vi "Prop Control Interface (Main).vi"() -> ()   [LabVIEW 2013]
uses:
  Common/State Machine.ctl
panel:
  out "Training Data":i32[][](array[numeric])
  out "Increment?":bool
  out "Sensor 4":T1(graph)
  out "Sensor 3":T1(graph)
  out "Sensor 2":T1(graph)
  in  "Frequency":u8(ring)=1 items=["CHAN0", "CHAN1", "CHAN2", "CHAN3", "CHAN4", "CHAN5"]
  in  "Threshold":u16=2047
  out "Readback":u8[](array[numeric])
  out "VISA Port":refnum<visa-resource-name>="COM4"
  out "baud rate":u32=921600
  out "data queue":refnum<queue>
  out "User Message":string
  out "MagPosSlider":dbl(slide) caption="Magnet Position" min=0.0 max=15.0 step=0.5 scale=0.0..15.0
  out "eTDS Connected?":bool
  out "Buffer":i32[][](array[numeric])
  out "Sensor 1":T1(graph)
  in  "Exit":bool
  in  "Start":bool
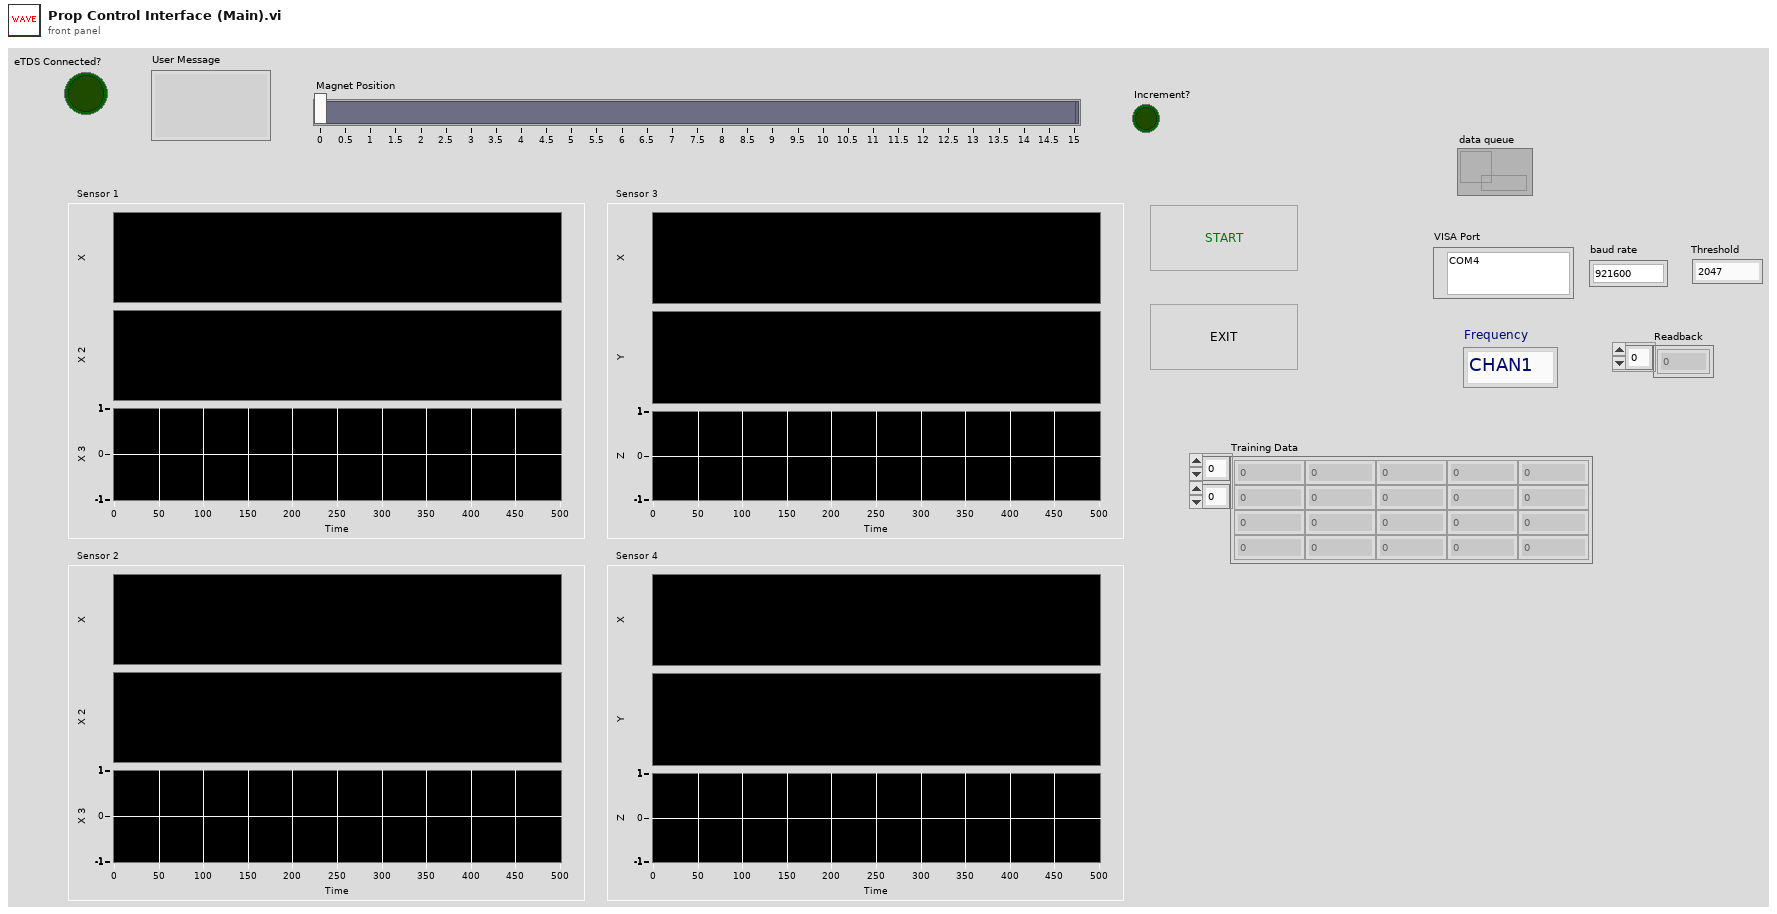
[diagram p1: front panel]
types:
  T1 = cluster{"Sensor 1[0]":i32, "Sensor 1[1]":i32, "Sensor 1[2]":i32}
  T2 = typedef "State Machine.ctl" = enum16{"Start", "Increment Slider", "Read Data", "Training SSP", "Stop"}
  T3 = enum8{"Enabled", "Disabled", "Disabled and Grayed Out"}
  T4 = cluster{"Sensor 1[0]":i32, "Sensor 1[1]":i32, "Sensor 1[2]":i32}[]
  T5 = cluster{"Sensor 4[0]":i32, "Sensor 4[1]":i32, "Sensor 4[2]":i32}
  T6 = cluster{"Sensor 3[0]":i32, "Sensor 3[1]":i32, "Sensor 3[2]":i32}
  T7 = cluster{"Sensor 2[0]":i32, "Sensor 2[1]":i32, "Sensor 2[2]":i32}
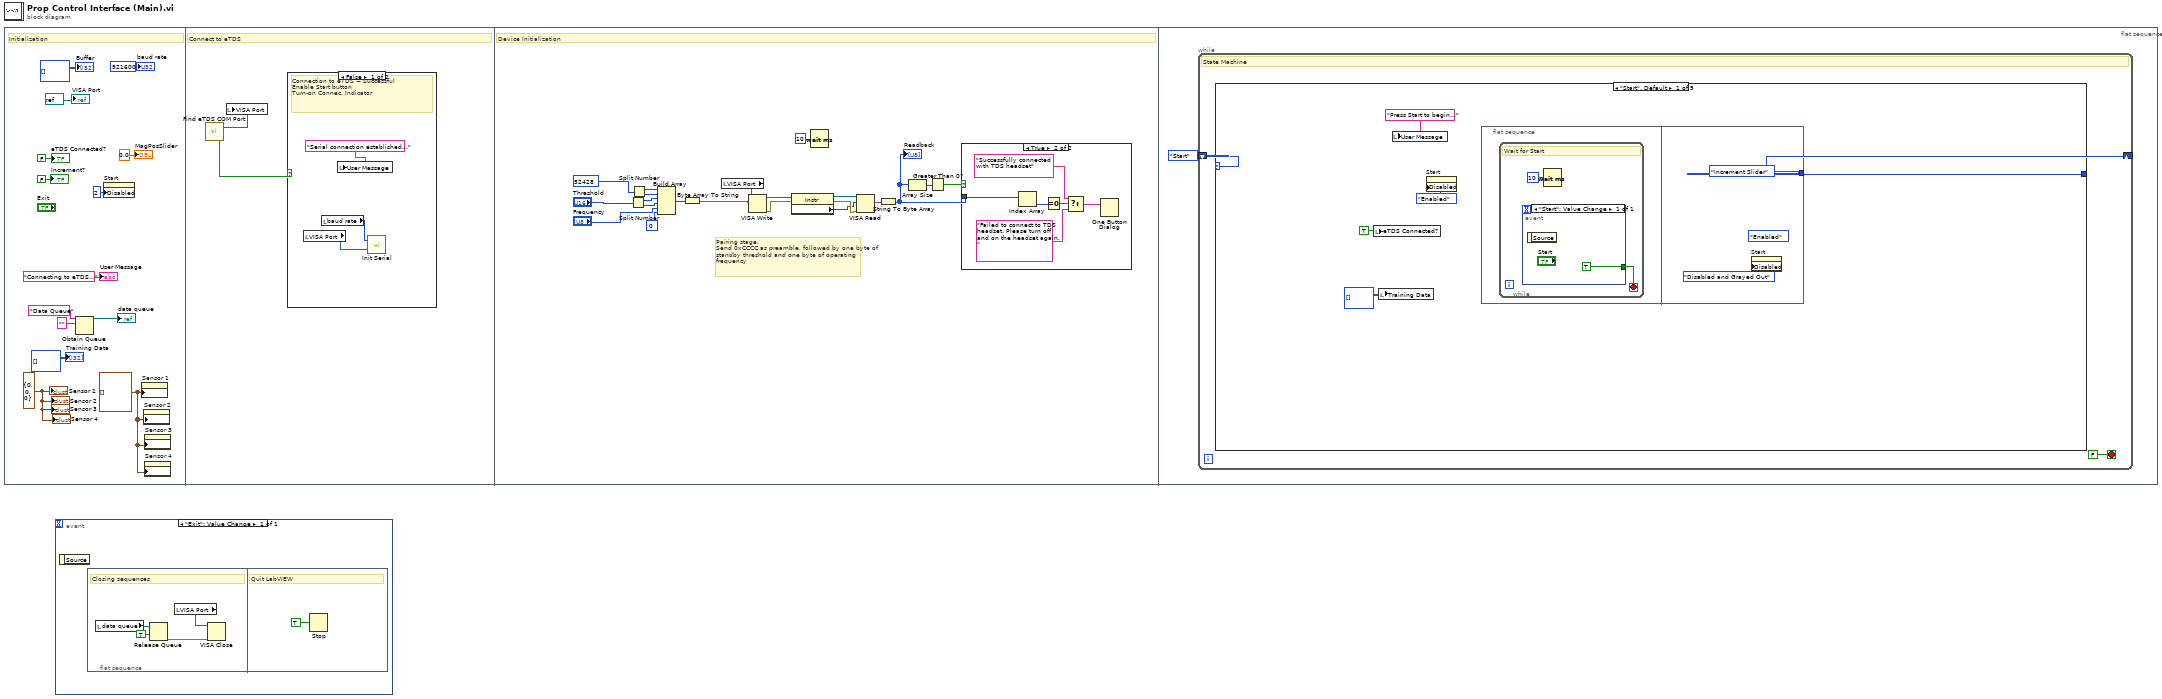
[diagram p0: block diagram]
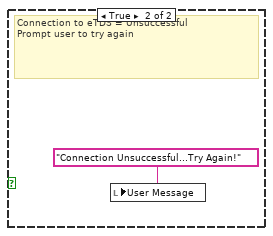
[diagram p2: hidden frame]
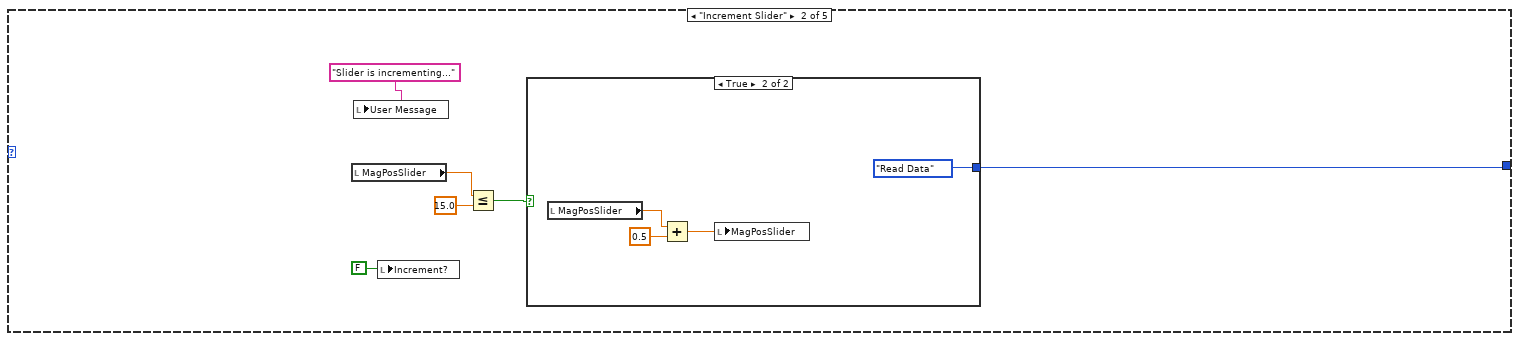
[diagram p4: hidden frame]
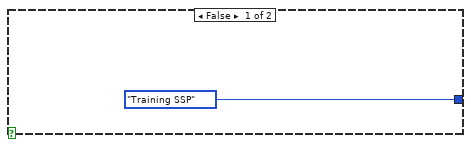
[diagram p5: hidden frame]
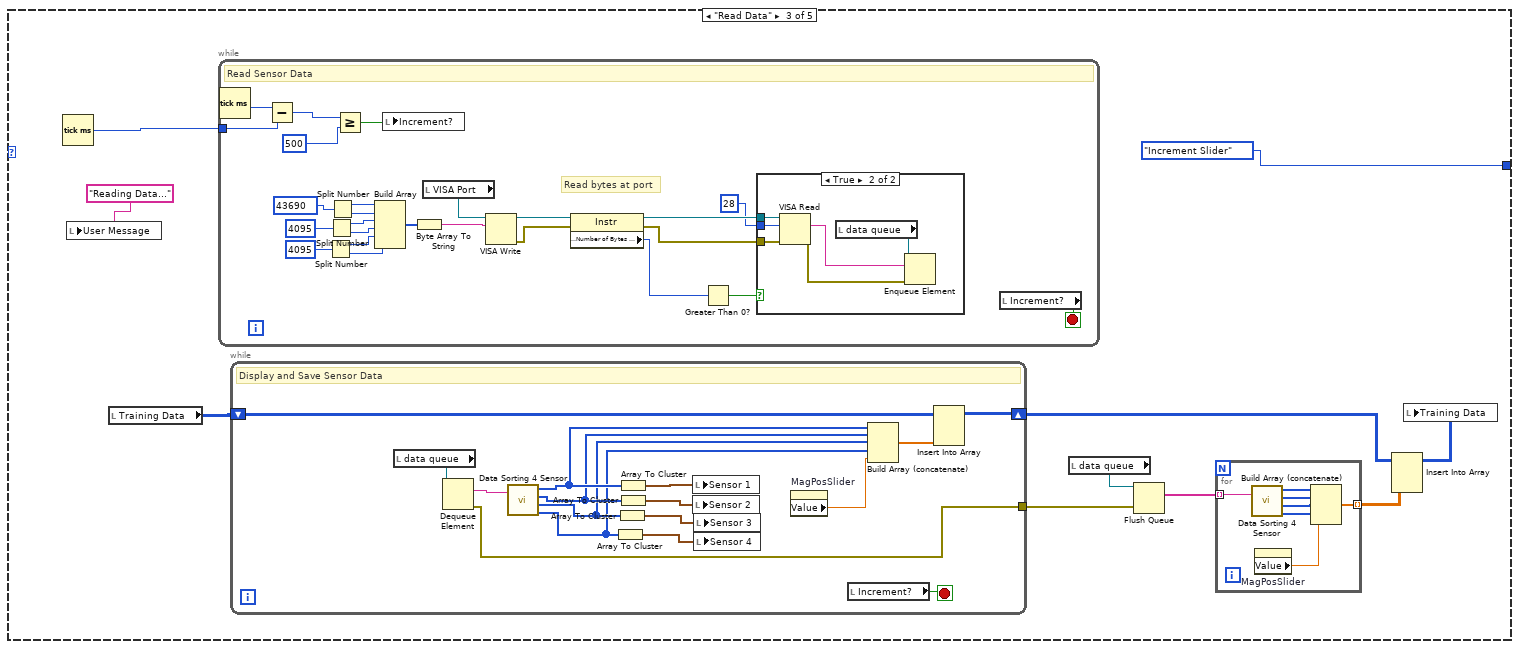
[diagram p6: hidden frame]
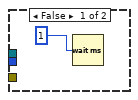
[diagram p7: hidden frame]
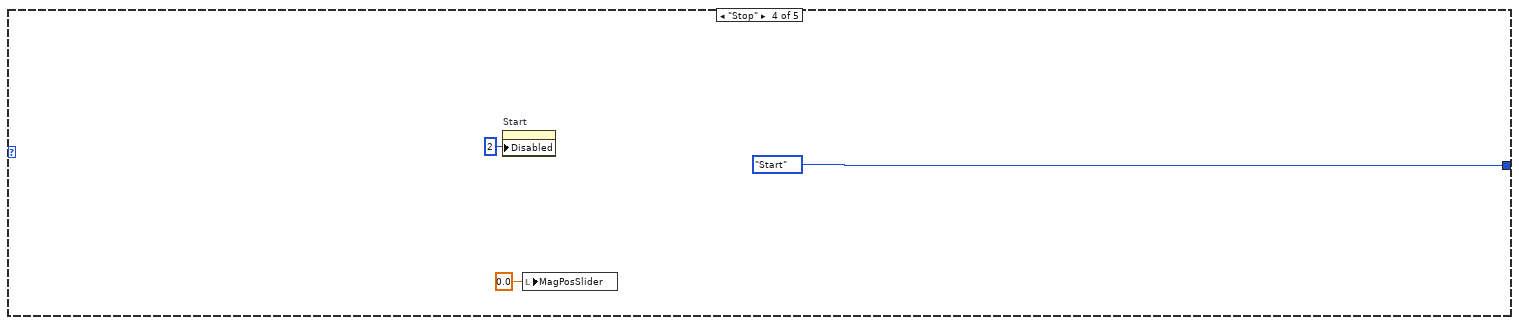
[diagram p8: hidden frame]
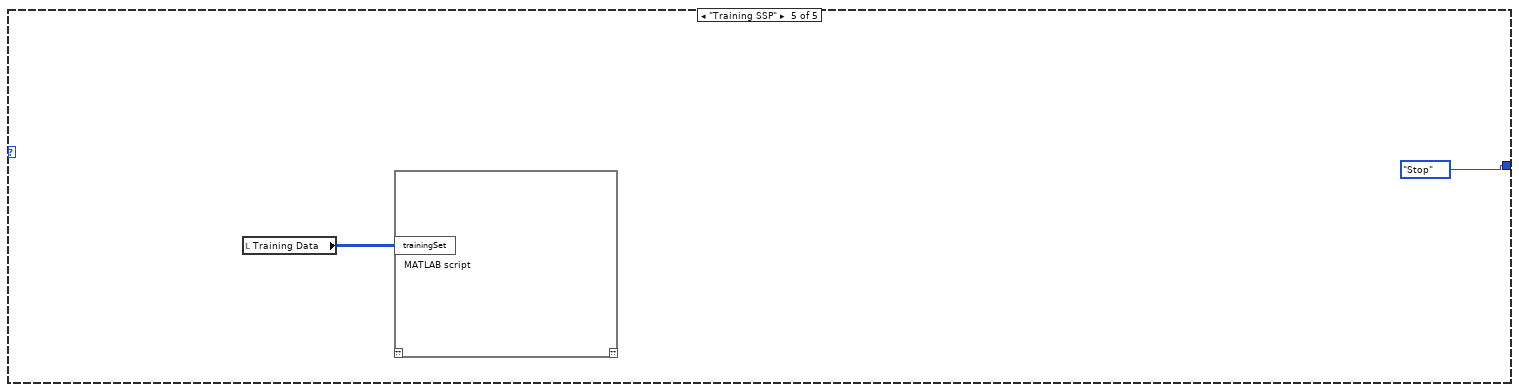
[diagram p9: hidden frame]
diagram:
  n1 = flat-sequence {
    frame #0 {
      w3 = T4 [] ("History Data")
      w4 = T1 {"Sensor 1[0]"=0, "Sensor 1[1]"=0, "Sensor 1[2]"=0} ("Sensor 1")
      # "Initialization"
      n2 = Obtain Queue(name (unnamed)="Data Queue" ("read buffer"), element data type="" ("read buffer")) -> (queue out=→"data queue":refnum<queue>)  [unwired: 3 in, 2 out]
      n3 = property on="Start" class="Bool"("Disabled"=u8 2) -> ()  [unwired: 2 in, 2 out]
      n4 = property on="Sensor 1" class="WFChart (strict)"("History Data"=w3) -> ()  [unwired: 2 in, 2 out]
      n5 = property on="Sensor 2" class="WFChart (strict)"("History Data"=w3) -> ()  [unwired: 2 in, 2 out]
      n6 = property on="Sensor 3" class="WFChart (strict)"("History Data"=w3) -> ()  [unwired: 2 in, 2 out]
      n7 = property on="Sensor 4" class="WFChart (strict)"("History Data"=w3) -> ()  [unwired: 2 in, 2 out]
      "eTDS Connected?" <- FALSE ("eTDS Connected?")
      "Buffer" <- i32[][] [] ("initialized array")
      "VISA Port" <- refnum<visa-resource-name> refnum ("VISA Resource Name")
      "baud rate" <- u32 921600 ("baud rate")
      "MagPosSlider" <- 0.0 ("MagPosSlider")
      "User Message" <- "Connecting to eTDS..." ("User Message")
      "Sensor 1" <- w4
      "Sensor 4" <- w4
      "Sensor 2" <- w4
      "Sensor 3" <- w4
      "Increment?" <- FALSE ("Increment?")
      "Training Data" <- i32[][] [] ("Training Data")
    }
    frame #1 {
      # "Connect to eTDS"
      n8 = call "Find eTDS COM Port.vi"() -> ("USB port"=w15:refnum<visa-resource-name>, "None/Multiple Device(s)?"=w16:bool)  [unwired: 1 in]
      n9 = local write "VISA Port"(w15) -> ()
      n10 = case shown="False" w16 {
        frame False {
          # "Connection to eTDS = Successful \nEnable Start button\nTurn-on Connec. Indicator"
          n11 = local read "VISA Port"() -> (w18:refnum<visa-resource-name>)
          n12 = local read "baud rate"() -> (w17:u32)
          n13 = local write "User Message"("Serial connection established..." ("User Message")) -> ()
          n14 = call "Init Serial.vi"("VISA resource name"=w18, "baud rate"=w17) -> ()  [unwired: 2 out]
        }
        frame True {
          # "Connection to eTDS = Unsuccessful\nPrompt user to try again"
          n15 = local write "User Message"("Connection Unsuccessful...Try Again!" ("User Message")) -> ()
        }
      }
    }
    frame #2 {
      # "Pairing stage.\nSend 0xCCCC as preamble, followed by one byte of standby threshold and one byte of operating frequency"
      # "Device Initialization"
      n16 = Split Number(x="Threshold") -> (hi(x)=w34:u8, lo(x)=w35:u8)
      n17 = Split Number(x=u16 52428 ("ChnA")) -> (hi(x)=w33:u8, lo(x)=w32:u8)
      n18 = Build Array(w33, w32, w34, w35, "Frequency", u8 0 ("ChnA")) -> (w31:u8[])
      n19 = Byte Array To String(unsigned byte array=w31) -> (string=w27:string)
      n20 = local read "VISA Port"() -> (w21:refnum<visa-resource-name>)
      n21 = VISA Write(VISA resource name=w21, write buffer=w27) -> (VISA resource name out=w25:refnum<visa-resource-name>, error out=w24:errorcluster)  [unwired: 1 in, 1 out]
      n22 = property class="Instr"(reference=w25, error in=w24) -> (reference out=w39:refnum<visa-resource-name>, error out=w38:errorcluster, "Serial Settings:Number of Bytes at Serial Port"=w36:u32)
      n23 = Wait (ms)(milliseconds to wait=u32 10) -> ()  [unwired: 1 out]
      n24 = VISA Read(VISA resource name=w39, byte count=w36, error in (no error)=w38) -> (read buffer=w37:string)  [unwired: 3 out]
      n25 = String To Byte Array(string=w37) -> (unsigned byte array=w26:u8[])
      "Readback" <- w26
      n26 = Array Size(array=w26) -> (size(s)=w40:i32)
      n27 = Greater Than 0?(x=w40) -> (x > 0?=w41:bool)
      n28 = case shown="True" w41 {
        tunnel: w26 -> [_ w43]
        frame False {
        }
        frame True {
          n29 = Index Array "Index Array"(array=w43) -> (element=w44:u8)  [unwired: 1 in]
          n30 = Equal To 0?(x=w44) -> (x = 0?=w42:bool)
          n31 = Select(t="Successfully connected with TDS headset", s=w42, f="Failed to connect to TDS headset. Please turn off and on the headset again.") -> (s? t:f=w47:string)
          n32 = One Button Dialog(message=w47) -> ()  [unwired: 1 in, 1 out]
        }
      }
    }
    frame #3 {
      n33 = while {
        shift-right: [w50] -> _
        shift-left: State_Machine."Start" -> [w49]
        stop <- FALSE stop-if-true
        # "State Machine"
        n34 = case shown="\"Start\", Default" w49 {
          tunnel: [w55 w65 State_Machine."Increment Slider" State_Machine."Start" State_Machine."Stop"] -> w50
          frame "Start", Default {
            n35 = local write "eTDS Connected?"(TRUE ("eTDS Connected?")) -> ()
            n36 = local write "Training Data"(i32[][] [] ("Training Data")) -> ()
            n37 = local write "User Message"("Press Start to begin..." ("User Message")) -> ()
            n38 = property on="Start" class="Bool"("Disabled"=T3."Enabled") -> ()  [unwired: 2 in, 2 out]
            n39 = flat-sequence {
              tunnel: [State_Machine."Increment Slider"] -> w55
              frame #0 {
                n40 = while {
                  stop <- w57 stop-if-true
                  # "Wait for Start"
                  n41 = event shown="[0] \"Start\": Value Change" {
                    selector: _ -> [_]
                    dyn-events: _ -> [_]
                    timeout: _ -> [_]
                    tunnel: [TRUE] -> w57
                    event "Start": Value Change {
                      n42 = event-data() -> ()  [unwired: 1 in, 1 out]
                    }
                  }
                  n43 = Wait (ms)(milliseconds to wait=u32 10) -> ()  [unwired: 1 out]
                }
              }
              frame #1 {
                (unwired) T3."Enabled" ("Disabled")
                n44 = property on="Start" class="Bool"("Disabled"=T3."Disabled and Grayed Out") -> ()  [unwired: 2 in, 2 out]
              }
            }
          }
          frame "Increment Slider" {
            n45 = local read "MagPosSlider"() -> (w67:dbl)
            n46 = local write "User Message"("Slider is incrementing..." ("User Message")) -> ()
            n47 = local write "Increment?"(FALSE ("Increment?")) -> ()
            n48 = Less Or Equal?(x=w67, y=15.0) -> (x <= y?=w63:bool)
            n49 = case shown="True" w63 {
              tunnel: [State_Machine."Training SSP" State_Machine."Read Data"] -> w65
              frame False {
              }
              frame True {
                n50 = local read "MagPosSlider"() -> (w71:dbl)
                n51 = Add(x=w71, y=0.5) -> (x+y=w70:dbl)
                n52 = local write "MagPosSlider"(w70) -> ()
              }
            }
          }
          frame "Read Data" {
            n53 = Tick Count (ms)() -> (millisecond timer value=w81:u32)
            n54 = local write "User Message"("Reading Data..." ("User Message")) -> ()
            n55 = local read "Training Data"() -> (w74:i32[][])
            n56 = while {
              tunnel: w81 -> [w110]
              stop <- w106 stop-if-true
              # "Read bytes at port"
              # "Read Sensor Data"
              n57 = Tick Count (ms)() -> (millisecond timer value=w111:u32)
              n58 = Subtract(x=w111, y=w110) -> (x-y=w109:u32)
              n59 = Split Number(x=u16 4095 ("ChnA")) -> (hi(x)=w117:u8, lo(x)=w116:u8)
              n60 = Split Number(x=u16 4095 ("ChnA")) -> (hi(x)=w122:u8, lo(x)=w123:u8)
              n61 = Split Number(x=u16 43690 ("ChnA")) -> (hi(x)=w121:u8, lo(x)=w120:u8)
              n62 = Greater Or Equal?(x=w109, y=u32 500 ("milliseconds to wait")) -> (x >= y?=w107:bool)
              n63 = Build Array(w121, w120, w122, w123, w117, w116) -> (w119:u8[])
              n64 = local write "Increment?"(w107) -> ()
              n65 = Byte Array To String(unsigned byte array=w119) -> (string=w118:string)
              n66 = local read "VISA Port"() -> (w112:refnum<visa-resource-name>)
              n67 = VISA Write(VISA resource name=w112, write buffer=w118) -> (VISA resource name out=w125:refnum<visa-resource-name>, error out=w124:errorcluster)  [unwired: 1 in, 1 out]
              n68 = property class="Instr"(reference=w125, error in=w124) -> (reference out=w129:refnum<visa-resource-name>, error out=w130:errorcluster, "Serial Settings:Number of Bytes at Serial Port"=w127:u32)
              n69 = Greater Than 0?(x=w127) -> (x > 0?=w128:bool)
              n70 = case shown="True" w128 {
                tunnel: w129 -> [_ w136]
                tunnel: w130 -> [_ w137]
                tunnel: u32 28 -> [_ w135]
                frame False {
                  n71 = Wait (ms)(milliseconds to wait=1) -> ()  [unwired: 1 out]
                }
                frame True {
                  n72 = VISA Read(VISA resource name=w136, byte count=w135, error in (no error)=w137) -> (read buffer=w134:string, error out=w133:errorcluster)  [unwired: 2 out]
                  n73 = local read "data queue"() -> (w132:refnum<queue>)
                  n74 = Enqueue Element(queue=w132, element=w134, error in (no error)=w133) -> ()  [unwired: 4 out]
                }
              }
              n75 = local read "Increment?"() -> (w106:bool)
            }
            n76 = while {
              shift-right: [w92] -> w76
              shift-left: w74 -> [w93]
              tunnel: [w90] -> w79
              stop <- w99 stop-if-true
              # "Display and Save Sensor Data"
              n77 = local read "data queue"() -> (w105:refnum<queue>)
              n78 = Dequeue Element(queue=w105) -> (element=w104:string, error out=w90:errorcluster)  [unwired: 1 in, 3 out]
              n79 = call "Data Sorting 4 Sensor.vi"("Data_Input"=w104) -> ("Sensor 1"=w98:i32[], "Sensor 2"=w97:i32[], "Sensor 3"=w96:i32[], "Sensor 4"=w95:i32[])  [unwired: 3 out]
              n80 = Array To Cluster(array=w95) -> (cluster=w100:T5)
              n81 = Array To Cluster(array=w96) -> (cluster=w101:T6)
              n82 = Array To Cluster(array=w98) -> (cluster=w103:T1)
              n83 = Array To Cluster(array=w97) -> (cluster=w102:T7)
              n84 = local write "Sensor 1"(w103) -> ()
              n85 = local write "Sensor 2"(w102) -> ()
              n86 = local write "Sensor 3"(w101) -> ()
              n87 = local write "Sensor 4"(w100) -> ()
              n88 = property on="MagPosSlider" class="Slide (strict)"() -> ("Value"=w91:dbl)  [unwired: 2 in, 2 out]
              n89 = local read "Increment?"() -> (w99:bool)
              n90 = Build Array (concatenate)(w98, w97, w96, w95, w91) -> (w94:dbl[])
              n91 = Insert Into Array(array=w93, new element=w94) -> (w92:i32[][])  [unwired: 2 in]
            }
            n92 = local read "data queue"() -> (w80:refnum<queue>)
            n93 = Flush Queue(queue=w80, error in (no error)=w79) -> (remaining elements=w78:string[])  [unwired: 2 out]
            n94 = for {
              tunnel: w78 -> [w89] mode=indexing
              tunnel: [w83] -> w77 mode=indexing
              n95 = call "Data Sorting 4 Sensor.vi"("Data_Input"=w89) -> ("Sensor 1"=w88:i32[], "Sensor 2"=w87:i32[], "Sensor 3"=w86:i32[], "Sensor 4"=w85:i32[])  [unwired: 3 out]
              n96 = property on="MagPosSlider" class="Slide (strict)"() -> ("Value"=w84:dbl)  [unwired: 2 in, 2 out]
              n97 = Build Array (concatenate)(w88, w87, w86, w85, w84) -> (w83:dbl[])
            }
            n98 = Insert Into Array(array=w76, new element=w77) -> (w75:i32[][])  [unwired: 2 in]
            n99 = local write "Training Data"(w75) -> ()
          }
          frame "Stop" {
            n100 = property on="Start" class="Bool"("Disabled"=u8 2) -> ()  [unwired: 2 in, 2 out]
            n101 = local write "MagPosSlider"(0.0 ("MagPosSlider")) -> ()
          }
          frame "Training SSP" {
            n102 = local read "Training Data"() -> (w142:i32[][])
            n103 = script code="MATLAB script"("trainingSet"=w142) -> ()  [unwired: 1 in, 1 out]
          }
        }
      }
    }
  }
  n104 = event shown="[0] \"Exit\": Value Change" {
    selector: _ -> [_]
    dyn-events: _ -> [_]
    timeout: _ -> [_]
    event "Exit": Value Change {
      n105 = event-data() -> ()  [unwired: 1 in, 1 out]
      n106 = flat-sequence {
        frame #0 {
          # "Closing sequences"
          n107 = local read "data queue"() -> (w145:refnum<queue>)
          n108 = Release Queue(queue=w145, force destroy? (F)=TRUE) -> (error out=w144:errorcluster)  [unwired: 1 in, 2 out]
          n109 = local read "VISA Port"() -> (w146:refnum<visa-resource-name>)
          n110 = VISA Close(VISA resource name=w146, error in (no error)=w144) -> ()  [unwired: 1 out]
        }
        frame #1 {
          # "Quit LabVIEW"
          n111 = Stop(stop? (T)=TRUE ("quit? (T)")) -> ()
        }
      }
    }
  }
